vi "auto_straight_mk1.vi"() -> ()   [LabVIEW 2012, in "BlockParty4150.lvrbt"]
uses:
  BlockParty4150.lvrbt
  <vilib>/NXT/Subs/LVHSConnector.ctl
  <vilib>/NXT/LegoClasses/BrickReference/BrickReference.lvclass
  <vilib>/NXT/Block Support/NXT_ButtonSelector.ctl
  <vilib>/NXT/Hardware/Plugins/Tetrix DC Motor/TetrixDCMotorAddress.ctl
  <vilib>/NXT/Hardware/Plugins/Tetrix 180 deg Servo/Tetrix180ServoAddress.ctl
  <vilib>/NXT/Dual Mode Library/Display/drawText.vi
  <vilib>/NXT/Dual Mode Library/Sound/Tone.vi
  <vilib>/NXT/NXTIO Xnodes/NXTIONodeSubVIs/TETRIX IO Move Servos.vi
  <vilib>/NXT/Dual Mode Library/Waits/Wait_Num(msec).vi
  <vilib>/NXT/Dual Mode Library/prims/inRangeAndCoerce/inRangeAndCoerce_int.vi
  <vilib>/NXT/Dual Mode Library/Display/drawNumber.vi
  <vilib>/NXT/NXTIO Xnodes/NXTIONodeSubVIs/TETRIX IO Move DC Motors.vi
  <vilib>/NXT/NXTIO Xnodes/NXTIONodeSubVIs/TETRIX IO Stop DC Motors.vi
  <vilib>/NXT/NXTIO Xnodes/AddressXNode/NXTIOAddress.xnode
  <vilib>/NXT/NXTIO Xnodes/NXTIOXNode/NXTIO.xnode
panel:
  out "Enabled":bool
  out "iter":i32
  out "NXT":T1
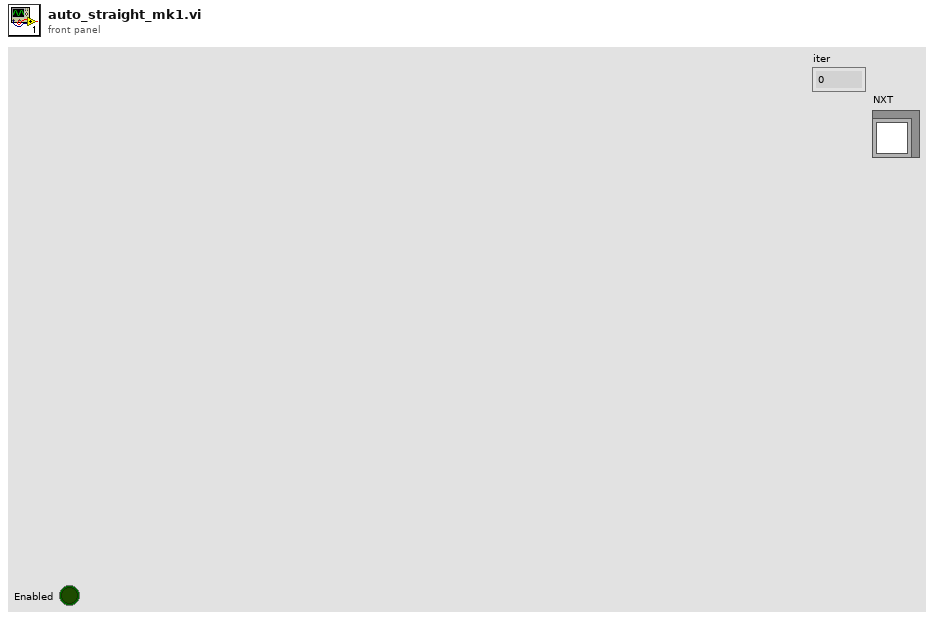
[diagram p1: front panel]
types:
  T1 = typedef "LVHSConnector.ctl" = refnum<class "BrickReference.lvclass">
  T2 = typedef "NXT_ButtonSelector.ctl" = u16
  T3 = typedef "Tetrix180ServoAddress.ctl" = i16
  T4 = typedef "TetrixDCMotorAddress.ctl" = i16
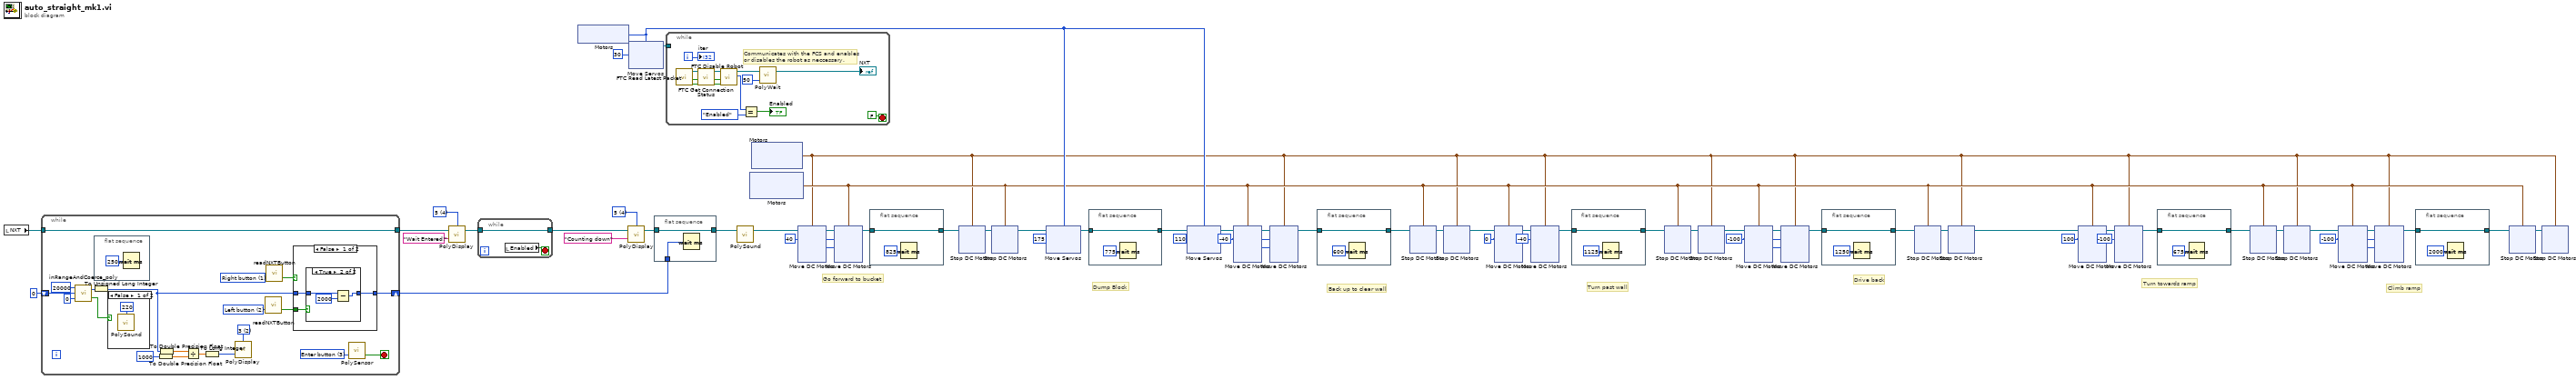
[diagram p0: block diagram]
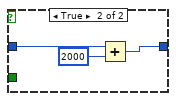
[diagram p4: hidden frame]
diagram:
  w8 = i16 4 items=["1", "2", "3", "4", "5", "6", "7", "8"] ("Line")
  w9 = i16 4 items=["1", "2", "3", "4", "5", "6", "7", "8"] ("Line")
  w20 = i8 -100 ("Power/Speed 1")
  w26 = i8 -100 ("Power/Speed 1")
  w25 = i8 100 ("Power/Speed 1")
  w30 = i8 -100 ("Power/Speed 1")
  w39 = i8 -40 ("Power/Speed 1")
  w41 = i8 0 ("Power/Speed 1")
  w48 = i8 -40 ("Power/Speed 1")
  w1 = i8 40 ("Power/Speed 1")
  # "Climb ramp"
  # "Drive back"
  # "Turn towards ramp"
  # "Turn past wall"
  # "Back up to clear wall"
  # "Dump Block"
  # "Go forward to bucket"
  n1 = local read "NXT"() -> (w2:T1)
  n2 = while {
    tunnel: [w80] -> w11
    tunnel: w2 -> [w80]
    shift-right: [w73] -> w12
    shift-left: u32 0 ("Power/Speed 1") -> [w66]
    stop <- w78 stop-if-true
    w72 = i16 2 items=["1", "2", "3", "4", "5", "6", "7", "8"] ("Line")
    w75 = T2 1 items=["Enter button"=3, "Left button"=2, "Right button"=1] ("Button (Enter button)")
    w74 = T2 2 items=["Enter button"=3, "Left button"=2, "Right button"=1] ("Button (Enter button)")
    w79 = T2 3 items=["Enter button"=3, "Left button"=2, "Right button"=1] ("Button (Enter button)")
    n3 = call-poly <vilib>:"inRangeAndCoerce_poly.vi"("lower limit"=0, "x"=w66, "upper limit"=20000) -> ("In Range?"=w61:bool, "coerced(x)"=w63:i32)
    n4 = To Unsigned Long Integer(number=w63) -> (unsigned 32bit integer=w62:u32)
    n5 = flat-sequence {
      frame #0 {
        n6 = Wait (ms)(milliseconds to wait=u32 250) -> ()  [unwired: 1 out]
      }
    }
    n7 = case shown="False" w61 {
      frame False {
        n8 = call-poly <vilib>:"PolySound.vi"("Tone (440 Hz)"=u16 220) -> ()  [unwired: 3 in, 1 out]
      }
      frame True {
      }
    }
    n9 = To Double Precision Float(number=u32 1000 ("Power/Speed 1")) -> (double precision float=w67:dbl)
    n10 = To Double Precision Float(number=w62) -> (double precision float=w69:dbl)
    n11 = Divide(x=w69, y=w67) -> (x/y=w70:dbl)
    n12 = To Long Integer(number=w70) -> (32bit integer=w68:i32)
    n13 = call-poly <vilib>:"PolyDisplay.vi"("number"=w68, "Line"=w72) -> ()  [unwired: 2 in, 1 out]
    n14 = call <vilib>:"readNXTButton.vi"("Button (Enter button)"=w74) -> ("Yes/No"=w77:bool)  [unwired: 2 in, 1 out]
    n15 = call <vilib>:"readNXTButton.vi"("Button (Enter button)"=w75) -> ("Yes/No"=w76:bool)  [unwired: 2 in, 1 out]
    n16 = case shown="False" w76 {
      tunnel: w77 -> [w85 _]
      tunnel: [w84 w91] -> w73
      tunnel: w62 -> [w83 w92]
      frame False {
        n17 = case shown="True" w85 {
          tunnel: [w86 w88] -> w84
          tunnel: w83 -> [w86 w89]
          frame False {
          }
          frame True {
            n18 = Subtract(x=w89, y=u32 2000) -> (x-y=w88:u32)
          }
        }
      }
      frame True {
        n19 = Add(x=w92, y=u32 2000) -> (x+y=w91:u32)
      }
    }
    n20 = call-poly <vilib>:"PolySensor.vi"("Button (Enter button)"=w79) -> ("Yes/No"=w78:bool)  [unwired: 2 in, 1 out]
  }
  n21 = call-poly <vilib>:"PolyDisplay.vi"("Text"="Wait Entered!", "NXT"=w11, "Line"=w9) -> ("NXT"=w5:T1)  [unwired: 1 in]
  n22 = while {
    tunnel: [w93] -> w4
    tunnel: w5 -> [w93]
    stop <- w94 stop-if-true
    n23 = local read "Enabled"() -> (w94:bool)
  }
  n24 = xnode "Motors"() -> ("Motor"=w50:T3)
  n25 = call-poly <vilib>:"PolyDisplay.vi"("Text"="Counting down", "NXT"=w4, "Line"=w8) -> ("NXT"=w6:T1)  [unwired: 1 in]
  n26 = xnode "Move Servos"("Position 1"=u8 30, "Servos"=w50) -> ("NXT"=w54:T1)  [unwired: 1 in]
  n27 = flat-sequence {
    tunnel: w6 -> [w96]
    tunnel: [w96] -> w14
    tunnel: w12 -> [w95]
    frame #0 {
      n28 = Wait (ms)(milliseconds to wait=w95) -> ()  [unwired: 1 out]
    }
  }
  n29 = while {
    tunnel: w54 -> [_]
    i -> [w98]
    stop <- FALSE stop-if-true
    # "Communicates with the FCS and enables \nor disables the robot as neccessary."
    n30 = call <vilib>:"FTC Read Latest Packet.vi"() -> ("Packet Received?"=w108:bool, "Stopped?"=w107:bool, "NXT"=w110:T1)  [unwired: 6 in, 3 out]
    n31 = call <vilib>:"FTC Get Connection Status.vi"("Packet Received?"=w108, "Stopped?"=w107, "NXT"=w110) -> ("Online?"=w100:bool, "Stopped?"=w101:bool, "NXT"=w109:T1)  [unwired: 5 in]
    n32 = call <vilib>:"FTC Disable Robot.vi"("Online?"=w100, "Stopped?"=w101, "NXT"=w109) -> ("Enabled?"=w104:enum16{"Disabled", "Enabled"}, "NXT"=w106:T1)  [unwired: 3 in]
    n33 = Equal?(x=w104, y=enum16{"Disabled", "Enabled"}."Enabled") -> (x = y?=→"Enabled":bool)
    n34 = call-poly <vilib>:"PolyWait.vi"("Time (100 msec)"=u32 50 ("Time (msec)"), "NXT"=w106) -> ("NXT"=→"NXT":T1)  [unwired: 2 in]
    "iter" <- w98
  }
  n35 = call-poly <vilib>:"PolySound.vi"("NXT"=w14) -> ("NXT"=w3:T1)  [unwired: 3 in]
  n36 = xnode "Motors"() -> ("Motor"=w28:cluster{"TetrixDCMotor":T4, "TetrixDCMotor":T4})
  n37 = xnode "Motors"() -> ("Motor"=w27:cluster{"TetrixDCMotor":T4, "TetrixDCMotor":T4})
  n38 = xnode "Move DC Motors"("Power/Speed 2"=w1, "Power/Speed 1"=w1, "Motors"=w27, "NXT"=w3) -> ("NXT"=w60:T1)
  n39 = xnode "Move DC Motors"("Power/Speed 2"=w1, "Power/Speed 1"=w1, "Motors"=w28, "NXT"=w60) -> ("NXT"=w59:T1)
  n40 = flat-sequence {
    tunnel: [w111] -> w58
    tunnel: w59 -> [w111]
    frame #0 {
      n41 = Wait (ms)(milliseconds to wait=u32 825) -> ()  [unwired: 1 out]
    }
  }
  n42 = xnode "Stop DC Motors"("Motors"=w27, "NXT"=w58) -> ("NXT"=w57:T1)
  n43 = xnode "Stop DC Motors"("Motors"=w28, "NXT"=w57) -> ("NXT"=w56:T1)
  n44 = xnode "Move Servos"("Position 1"=u8 175, "Servos"=w50, "NXT"=w56) -> ("NXT"=w52:T1)
  n45 = flat-sequence {
    tunnel: [w113] -> w51
    tunnel: w52 -> [w113]
    frame #0 {
      n46 = Wait (ms)(milliseconds to wait=u32 775) -> ()  [unwired: 1 out]
    }
  }
  n47 = xnode "Move Servos"("Position 1"=u8 110, "Servos"=w50, "NXT"=w51) -> ("NXT"=w47:T1)
  n48 = xnode "Move DC Motors"("Power/Speed 2"=w48, "Power/Speed 1"=w48, "Motors"=w28, "NXT"=w47) -> ("NXT"=w45:T1)
  n49 = xnode "Move DC Motors"("Power/Speed 2"=w48, "Power/Speed 1"=w48, "Motors"=w27, "NXT"=w45) -> ("NXT"=w46:T1)
  n50 = flat-sequence {
    tunnel: [w115] -> w43
    tunnel: w46 -> [w115]
    frame #0 {
      n51 = Wait (ms)(milliseconds to wait=u32 600) -> ()  [unwired: 1 out]
    }
  }
  n52 = xnode "Stop DC Motors"("Motors"=w28, "NXT"=w43) -> ("NXT"=w44:T1)
  n53 = xnode "Stop DC Motors"("Motors"=w27, "NXT"=w44) -> ("NXT"=w40:T1)
  n54 = xnode "Move DC Motors"("Power/Speed 2"=w41, "Power/Speed 1"=w41, "Motors"=w28, "NXT"=w40) -> ("NXT"=w42:T1)
  n55 = xnode "Move DC Motors"("Power/Speed 2"=w39, "Power/Speed 1"=w39, "Motors"=w27, "NXT"=w42) -> ("NXT"=w36:T1)
  n56 = flat-sequence {
    tunnel: [w117] -> w38
    tunnel: w36 -> [w117]
    frame #0 {
      n57 = Wait (ms)(milliseconds to wait=u32 1125) -> ()  [unwired: 1 out]
    }
  }
  n58 = xnode "Stop DC Motors"("Motors"=w28, "NXT"=w38) -> ("NXT"=w37:T1)
  n59 = xnode "Stop DC Motors"("Motors"=w27, "NXT"=w37) -> ("NXT"=w31:T1)
  n60 = xnode "Move DC Motors"("Power/Speed 2"=w30, "Power/Speed 1"=w30, "Motors"=w28, "NXT"=w31) -> ("NXT"=w32:T1)
  n61 = xnode "Move DC Motors"("Power/Speed 2"=w30, "Power/Speed 1"=w30, "Motors"=w27, "NXT"=w32) -> ("NXT"=w35:T1)
  n62 = flat-sequence {
    tunnel: [w119] -> w33
    tunnel: w35 -> [w119]
    frame #0 {
      n63 = Wait (ms)(milliseconds to wait=u32 1250) -> ()  [unwired: 1 out]
    }
  }
  n64 = xnode "Stop DC Motors"("Motors"=w28, "NXT"=w33) -> ("NXT"=w34:T1)
  n65 = xnode "Stop DC Motors"("Motors"=w27, "NXT"=w34) -> ("NXT"=w29:T1)
  n66 = xnode "Move DC Motors"("Power/Speed 2"=w25, "Power/Speed 1"=w25, "Motors"=w28, "NXT"=w29) -> ("NXT"=w24:T1)
  n67 = xnode "Move DC Motors"("Power/Speed 2"=w26, "Power/Speed 1"=w26, "Motors"=w27, "NXT"=w24) -> ("NXT"=w21:T1)
  n68 = flat-sequence {
    tunnel: [w121] -> w23
    tunnel: w21 -> [w121]
    frame #0 {
      n69 = Wait (ms)(milliseconds to wait=u32 675) -> ()  [unwired: 1 out]
    }
  }
  n70 = xnode "Stop DC Motors"("Motors"=w28, "NXT"=w23) -> ("NXT"=w22:T1)
  n71 = xnode "Stop DC Motors"("Motors"=w27, "NXT"=w22) -> ("NXT"=w15:T1)
  n72 = xnode "Move DC Motors"("Power/Speed 2"=w20, "Power/Speed 1"=w20, "Motors"=w28, "NXT"=w15) -> ("NXT"=w19:T1)
  n73 = xnode "Move DC Motors"("Power/Speed 2"=w20, "Power/Speed 1"=w20, "Motors"=w27, "NXT"=w19) -> ("NXT"=w16:T1)
  n74 = flat-sequence {
    tunnel: [w123] -> w18
    tunnel: w16 -> [w123]
    frame #0 {
      n75 = Wait (ms)(milliseconds to wait=u32 2000) -> ()  [unwired: 1 out]
    }
  }
  n76 = xnode "Stop DC Motors"("Motors"=w28, "NXT"=w18) -> ("NXT"=w17:T1)
  n77 = xnode "Stop DC Motors"("Motors"=w27, "NXT"=w17) -> ()  [unwired: 1 out]
